vi "CSV SENDER 2.vi"() -> ()   [LabVIEW 2021]
panel:
  out "Waveform Graph 10":dynamicdata(graph)
  out "Numeric 3":dbl
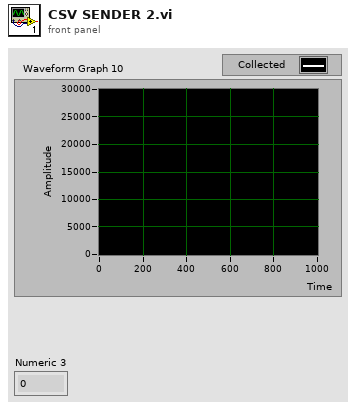
[diagram p1: front panel]
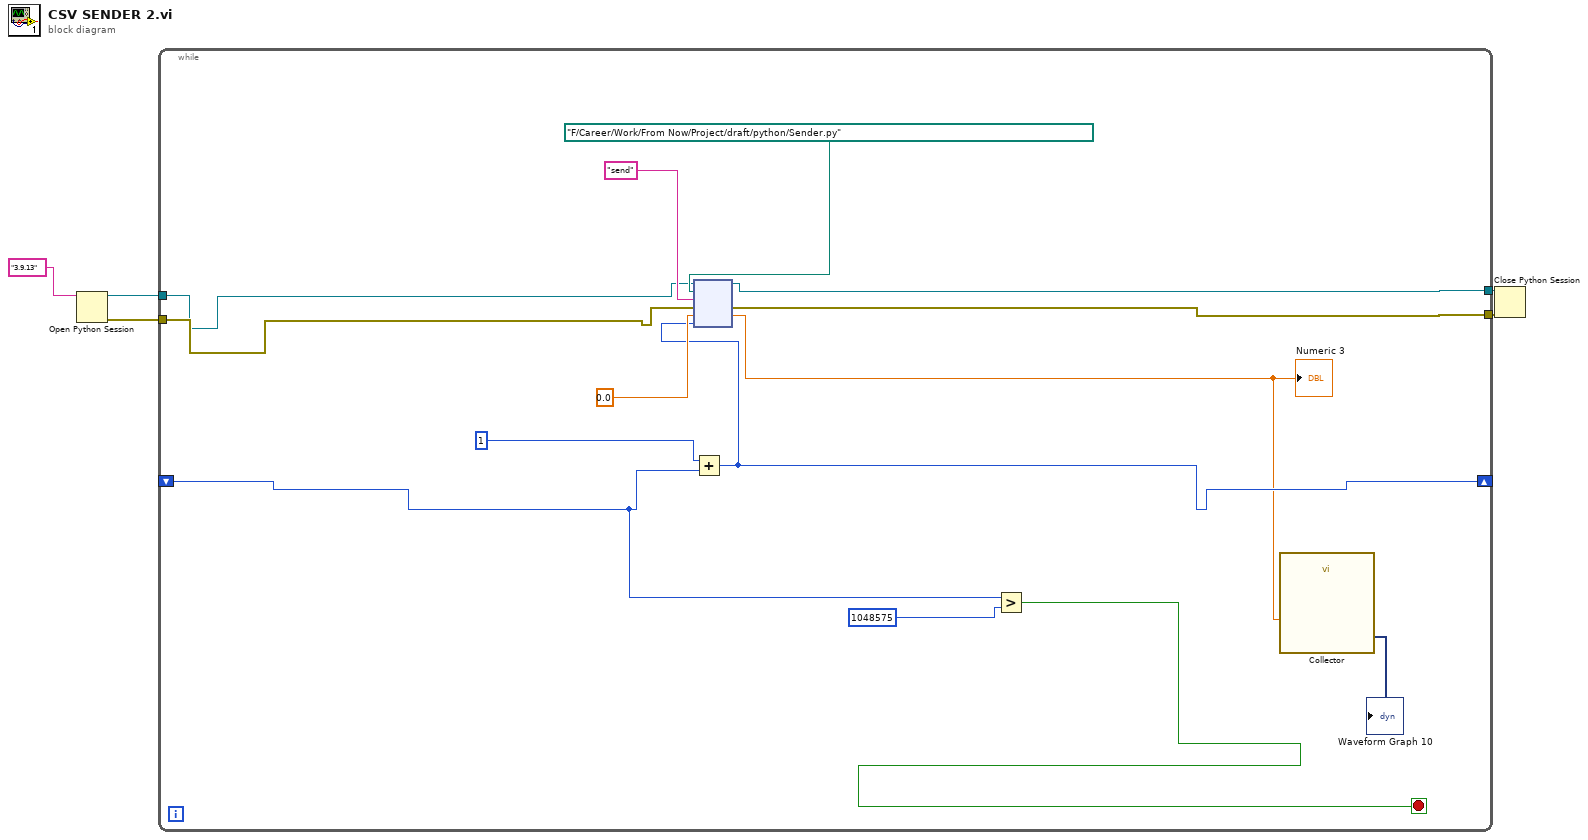
[diagram p0: block diagram]
diagram:
  n1 = Open Python Session(python version="3.9.13" ("Python version")) -> (session out=w4:refnum<k35>, error out=w3:errorcluster)  [unwired: 2 in]
  n2 = while {
    tunnel: w4 -> [w11]
    tunnel: w3 -> [w12]
    tunnel: [w14] -> w2
    tunnel: [w13] -> w1
    shift-right: [w8] -> _
    shift-left: _ -> [w9]
    stop <- w10 stop-if-true
    n3 = Add(x=1, y=w9) -> (x+y=w8:i32)
    n4 = node(w11, path "F:/Career/Work/From Now/Project/draft/python/Sender.py" ("module path"), "send" ("function name"), w12, 0.0, w8) -> (w14:refnum<k35>, w13:errorcluster, w7:dbl)  [unwired: 1 in, 2 out]
    "Numeric 3" <- w7
    n5 = Greater?(x=w9, y=1048575) -> (0:w10:bool)
    n6 = call "Collector"("Signals"=w7) -> ("Collected Signals"=→"Waveform Graph 10":dynamicdata)  [unwired: 9 in, 1 out]
  }
  n7 = Close Python Session(session in=w2, error in=w1) -> ()  [unwired: 1 out]
